vi "Average3.vi"() -> ()   [LabVIEW 2016]
panel:
  out "average":dbl
  in  "3":dbl
  in  "2":dbl
  in  "1":dbl
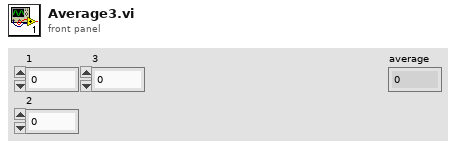
[diagram p1: front panel]
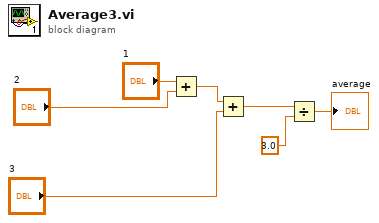
[diagram p0: block diagram]
diagram:
  n1 = Add(x="1", y="2") -> (x+y=w7:dbl)
  n2 = Add(x=w7, y="3") -> (x+y=w3:dbl)
  n3 = Divide(x=w3, y=3.0) -> (x/y=→"average":dbl)
